vi "EstimateTargetingInformation.vi"(0 "Robot X (in)":dbl, 1 "Robot Y (in)":dbl) -> (2 "Estimated Distance to Target (in)":dbl, 3 "Estimated Robot Heading to Target (deg)":dbl, 4 "Estimated Turret Heading to Target (deg)":dbl)   [LabVIEW 2019]
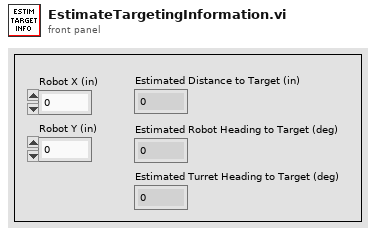
[diagram p1: front panel]
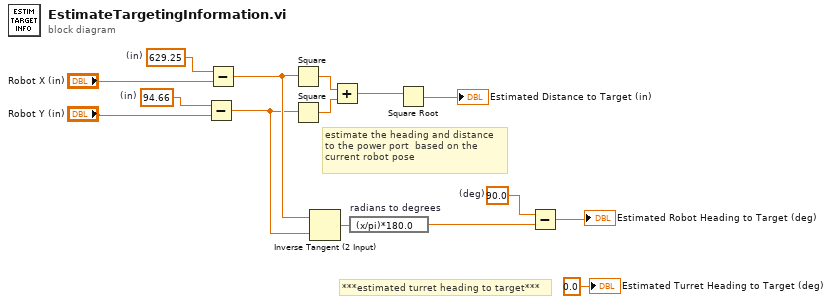
[diagram p0: block diagram]
diagram:
  w6 = 90.0  # (deg)
  w9 = 94.66  # (in)
  w11 = 629.25  # (in)
  # "***estimated turret heading to target***"
  # "estimate the heading and distance\nto the power port  based on the\ncurrent robot pose"
  n1 = Subtract(x=w9, y="Robot Y (in)") -> (x-y=w7:dbl)
  n2 = Subtract(x=w11, y="Robot X (in)") -> (x-y=w8:dbl)
  n3 = Square(x=w8) -> (x^2=w15:dbl)
  n4 = Square(x=w7) -> (x^2=w14:dbl)
  n5 = Inverse Tangent (2 Input)(1:w7, 2:w8) -> (0:w4:dbl)
  n6 = Add(x=w15, y=w14) -> (x+y=w13:dbl)
  n7 = expression code="(x/pi)*180.0" "radians to degrees"(w4) -> (w3:dbl)
  n8 = Square Root(x=w13) -> (sqrt(x)=→"Estimated Distance to Target (in)":dbl)
  n9 = Subtract(x=w6, y=w3) -> (x-y=→"Estimated Robot Heading to Target (deg)":dbl)
  "Estimated Turret Heading to Target (deg)" <- 0.0 ("Estimated Turret Heading to Target (deg)")
